vi "ADC_and_DAC.vi"(1 "ADS Mode In":i32=1 min=1 max=6 step=1, 2 "Board address":i32=4660 format="%x") -> (0 "ADS Mode Out":i32)   [LabVIEW 2011]
doc: "This VI is a pop-up window that allows full access to the MUX, DAC, and A/D converter. This should be included with all USB-DAQ applications as a debug tool. You can also look through the software as an example of how to configure the MUX, DAC, and A/D converter."
panel:
  out "ADC 2":string
  out "ADC 1":string
  in  "User Ref Voltage":dbl
  in  "Connect I Loop Readback":bool
  in  "ADS2- MUX":enum32{"Open", "Dac C", "GND"}(radio)
  in  "ADS2+ MUX":enum32{"Open", "Dac D", "GND"}(radio)
  in  "ADS1- MUX":enum32{"Open", "Dac A", "GND"}(radio)
  in  "ADS1+ MUX":enum32{"Open", "Dac B", "GND"}(radio)
  in  "ReadADC_2":bool
  in  "ReadADC_1":bool
  in  "Write_DAC_D":bool
  in  "Write_DAC_C":bool
  in  "Write_DAC_B":bool
  in  "Write_DAC_A":bool
  in  "DAC_D":dbl=0.017 min=0.017 max=5.0
  in  "DAC_C":dbl=0.017 min=0.017 max=5.0
  in  "DAC_B":dbl=0.017 min=0.017 max=5.0
  in  "DAC_A":dbl=0.017 min=0.017 max=5.0
  in  "ADC Config":T1(radio)
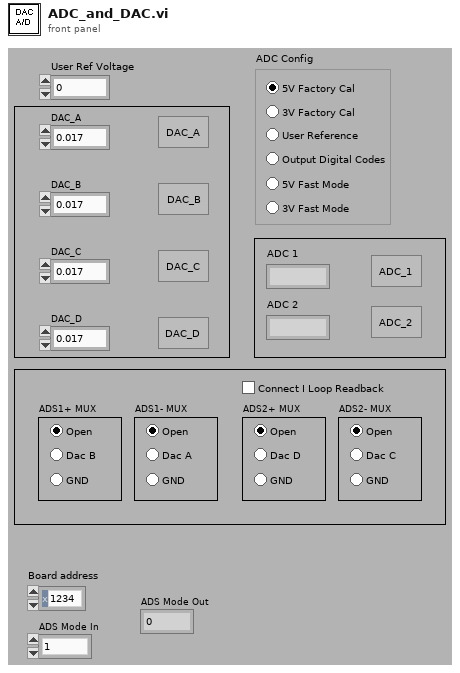
[diagram p1: front panel]
types:
  T1 = enum32{"5V Factory Cal", "3V Factory Cal", "User Reference", "Output Digital Codes", "5V Fast Mode", "3V Fast Mode"}
  T2 = enum32{"Invalid", "Standard", "Closed", "Hidden", "Minimized", "Maximized"}
  T3 = enum16{"Always On", "Always Off", "Off While Running"}
  T4 = enum32{"invalid app kind", "Development System", "Run Time System", "Student Edition", "Embedded LabVIEW", "Evaluation", "Custom"}
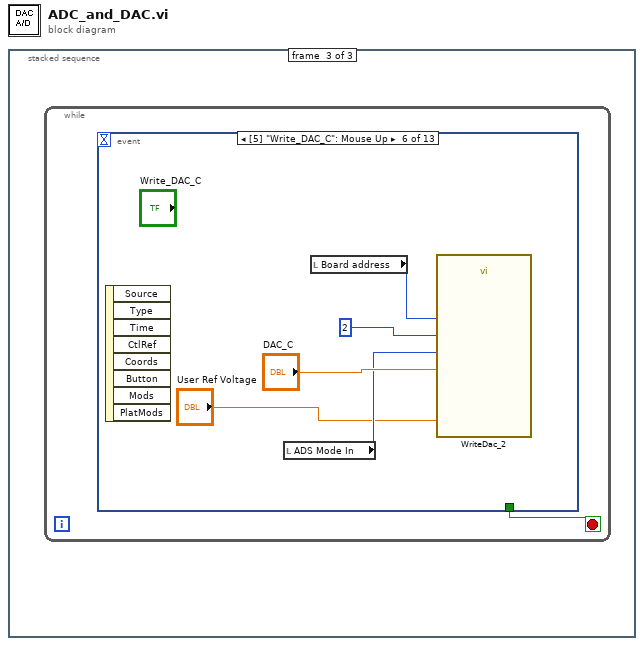
[diagram p0: block diagram]
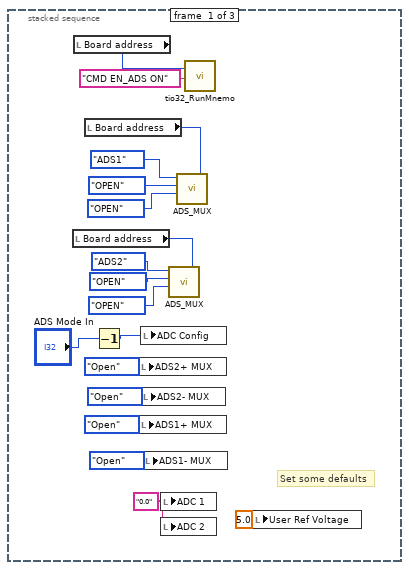
[diagram p2: hidden frame]
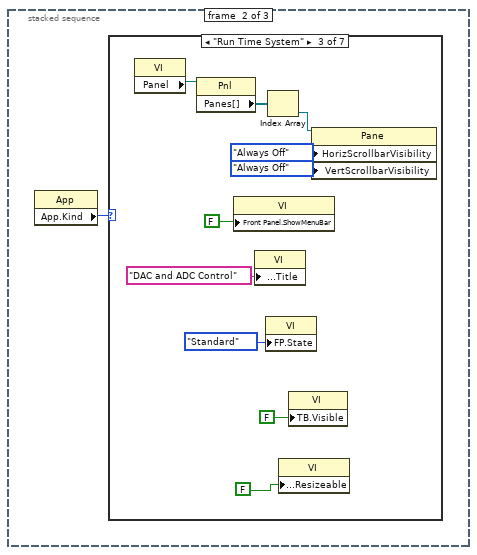
[diagram p3: hidden frame]
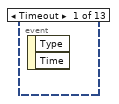
[diagram p10: hidden frame]
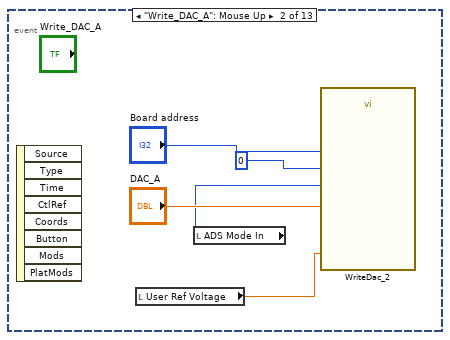
[diagram p11: hidden frame]
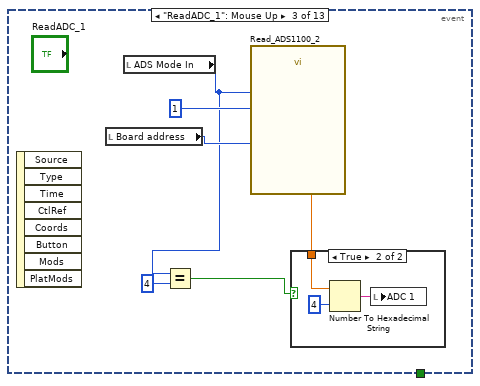
[diagram p12: hidden frame]
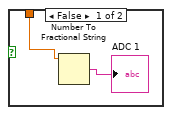
[diagram p13: hidden frame]
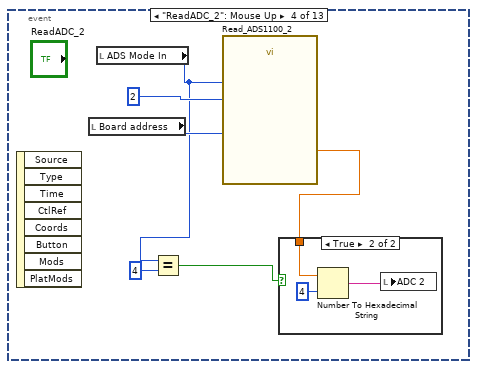
[diagram p14: hidden frame]
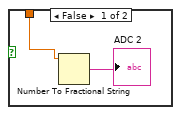
[diagram p15: hidden frame]
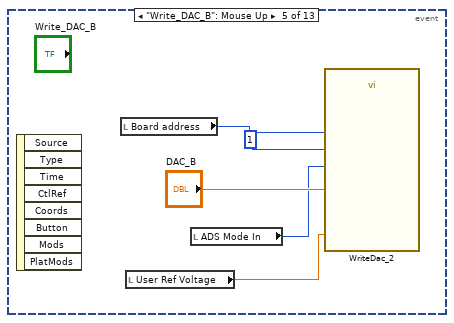
[diagram p16: hidden frame]
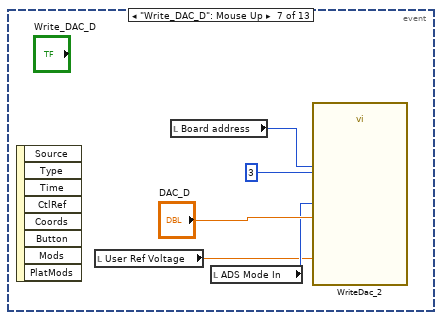
[diagram p17: hidden frame]
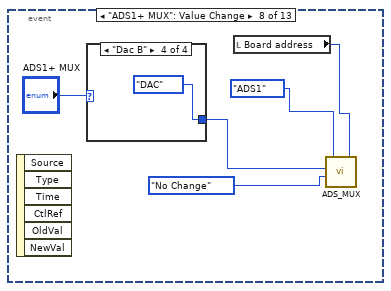
[diagram p18: hidden frame]
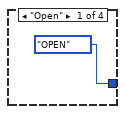
[diagram p19: hidden frame]
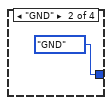
[diagram p20: hidden frame]
diagram:
  n1 = stacked-sequence {
    frame #0 {
      w2 = "0.0" ("ADC 1")
      # "Set some defaults"
      n2 = local read "Board address"() -> (w8:i32)
      n3 = local read "Board address"() -> (w18:i32)
      n4 = local read "Board address"() -> (w9:i32)
      n5 = Decrement(x="ADS Mode In") -> (x-1=w3:i32)
      n6 = local write "ADS2+ MUX"(enum32{"Open", "Dac D", "GND"}."Open" ("ADS2+ MUX")) -> ()
      n7 = local write "ADS1+ MUX"(enum32{"Open", "Dac B", "GND"}."Open" ("ADS1+ MUX")) -> ()
      n8 = local write "ADC Config"(w3) -> ()
      n9 = local write "ADS2- MUX"(enum32{"Open", "Dac C", "GND"}."Open" ("ADS2- MUX")) -> ()
      n10 = local write "ADS1- MUX"(enum32{"Open", "Dac A", "GND"}."Open" ("ADS1- MUX")) -> ()
      n11 = local write "ADC 1"(w2) -> ()
      n12 = local write "ADC 2"(w2) -> ()
      n13 = call "ADS_MUX.vi"("Board address"=w8, "In Neg"=enum16{"OPEN", "GND", "DAC", "No Change"}."OPEN", "In Pos"=enum16{"OPEN", "GND", "DAC", "No Change"}."OPEN", "Mux Num"=enum16{"ADS1", "ADS2"}."ADS2") -> ()  [unwired: 1 in, 1 out]
      n14 = call "ADS_MUX.vi"("Board address"=w9, "In Neg"=enum16{"OPEN", "GND", "DAC", "No Change"}."OPEN", "In Pos"=enum16{"OPEN", "GND", "DAC", "No Change"}."OPEN", "Mux Num"=enum16{"ADS1", "ADS2"}."ADS1") -> ()  [unwired: 1 in, 1 out]
      n15 = call "tio32_RunMnemo.vi"("Device address"=w18, "command string"="CMD EN_ADS ON") -> ()  [unwired: 7 in, 11 out]
      n16 = local write "User Ref Voltage"(5.0 ("User Ref Voltage")) -> ()
    }
    frame #1 {
      n17 = property class="App"() -> ("App.Kind"=w19:T4)  [unwired: 2 in, 2 out]
      n18 = case shown="\"Run Time System\"" w19 {
        frame "invalid app kind", Default {
        }
        frame "Development System" {
        }
        frame "Run Time System" {
          n19 = property class="VI"() -> ("Panel"=w29:refnum<vi>)  [unwired: 2 in, 2 out]
          n20 = property class="Pnl"(reference=w29) -> ("Panes[]"=w28:refnum<vi>[])  [unwired: 1 in, 2 out]
          n21 = property class="VI"("Front Panel.ShowMenuBar"=FALSE ("Front Panel Window:Show Menu Bar")) -> ()  [unwired: 2 in, 2 out]
          n22 = property class="VI"("Front Panel.Title"="DAC and ADC Control" ("Front Panel Window:Title")) -> ()  [unwired: 2 in, 2 out]
          n23 = property class="VI"("FP.State"=T2."Standard" ("Front Panel Window:State")) -> ()  [unwired: 2 in, 2 out]
          n24 = Index Array(array=w28) -> (element=w27:refnum<vi>)  [unwired: 1 in]
          n25 = property class="VI"("Front Panel.Resizeable"=FALSE ("Front Panel Window:Resizeable")) -> ()  [unwired: 2 in, 2 out]
          n26 = property class="VI"("TB.Visible"=FALSE ("Front Panel Window:Resizeable")) -> ()  [unwired: 2 in, 2 out]
          n27 = property class="Pane"(reference=w27, "HorizScrollbarVisibility"=T3."Always Off" ("Horizontal Scrollbar Visibility"), "VertScrollbarVisibility"=T3."Always Off" ("Vertical Scrollbar Visibility")) -> ()  [unwired: 1 in, 2 out]
        }
        frame "Student Edition" {
        }
        frame "Embedded LabVIEW" {
        }
        frame "Evaluation" {
        }
        frame "Custom" {
        }
      }
    }
    frame #2 {
      n28 = while {
        stop <- w30 stop-if-true
        n29 = event shown="[5] \"Write_DAC_C\": Mouse Up" {
          selector: _ -> [_ _ _ _ _ _ _ _ _ _ _ _ _]
          dyn-events: _ -> [_ _ _ _ _ _ _ _ _ _ _ _ _]
          timeout: _ -> [_ _ _ _ _ _ _ _ _ _ _ _ _]
          tunnel: [_ _ _ _ _ _ _ _ _ _ _ _ w116] -> w30
          event Timeout {
            n30 = event-data() -> ()  [unwired: 1 in, 2 out]
          }
          event "Write_DAC_A": Mouse Up {
            n31 = event-data() -> ()  [unwired: 1 in, 8 out]
            n32 = local read "User Ref Voltage"() -> (w31:dbl)
            n33 = local read "ADS Mode In"() -> (w32:i32)
            n34 = call "WriteDac_2.vi"("ref"=w31, "value"="DAC_A", "mode"=w32, "DAC number"=0, "Board address"="Board address") -> ()  [unwired: 4 in, 1 out]
          }
          event "ReadADC_1": Mouse Up {
            n35 = event-data() -> ()  [unwired: 1 in, 8 out]
            n36 = local read "Board address"() -> (w41:i32)
            n37 = local read "ADS Mode In"() -> (w38:i32)
            n38 = Equal?(x=w38, y=4) -> (x = y?=w36:bool)
            n39 = call "Read_ADS1100_2.vi"("USB DAQ Address"=w41, "ADS Mode"=w38, "ADS number"=1 ("mode")) -> ("ADC"=w39:dbl)  [unwired: 1 in, 1 out]
            n40 = case shown="True" w36 {
              tunnel: w39 -> [w43 w46]
              frame False {
                n41 = Number To Fractional String(number=w43) -> (F-format string=→"ADC 1":string)  [unwired: 3 in]
              }
              frame True {
                n42 = Number To Hexadecimal String(1:i16 4 ("width (-)"), 2:w46) -> (0:w45:string)
                n43 = local write "ADC 1"(w45) -> ()
              }
            }
          }
          event "ReadADC_2": Mouse Up {
            n44 = event-data() -> ()  [unwired: 1 in, 8 out]
            n45 = local read "Board address"() -> (w51:i32)
            n46 = local read "ADS Mode In"() -> (w47:i32)
            n47 = Equal?(x=w47, y=4) -> (x = y?=w49:bool)
            n48 = call "Read_ADS1100_2.vi"("USB DAQ Address"=w51, "ADS Mode"=w47, "ADS number"=2) -> ("ADC"=w48:dbl)  [unwired: 1 in, 1 out]
            n49 = case shown="True" w49 {
              tunnel: w48 -> [w54 w57]
              frame False {
                n50 = Number To Fractional String(number=w54) -> (F-format string=→"ADC 2":string)  [unwired: 3 in]
              }
              frame True {
                n51 = Number To Hexadecimal String(1:i16 4 ("width (-)"), 2:w57) -> (0:w55:string)
                n52 = local write "ADC 2"(w55) -> ()
              }
            }
          }
          event "Write_DAC_B": Mouse Up {
            n53 = event-data() -> ()  [unwired: 1 in, 8 out]
            n54 = local read "Board address"() -> (w62:i32)
            n55 = local read "User Ref Voltage"() -> (w58:dbl)
            n56 = local read "ADS Mode In"() -> (w59:i32)
            n57 = call "WriteDac_2.vi"("ref"=w58, "value"="DAC_B", "mode"=w59, "DAC number"=1, "Board address"=w62) -> ()  [unwired: 4 in, 1 out]
          }
          event "Write_DAC_C": Mouse Up {
            n58 = event-data() -> ()  [unwired: 1 in, 8 out]
            n59 = local read "ADS Mode In"() -> (w64:i32)
            n60 = local read "Board address"() -> (w67:i32)
            n61 = call "WriteDac_2.vi"("ref"="User Ref Voltage", "value"="DAC_C", "mode"=w64, "DAC number"=2, "Board address"=w67) -> ()  [unwired: 4 in, 1 out]
          }
          event "Write_DAC_D": Mouse Up {
            n62 = event-data() -> ()  [unwired: 1 in, 8 out]
            n63 = local read "User Ref Voltage"() -> (w68:dbl)
            n64 = local read "Board address"() -> (w70:i32)
            n65 = local read "ADS Mode In"() -> (w69:i32)
            n66 = call "WriteDac_2.vi"("ref"=w68, "value"="DAC_D", "mode"=w69, "DAC number"=3, "Board address"=w70) -> ()  [unwired: 4 in, 1 out]
          }
          event "ADS1+ MUX": Value Change {
            n67 = event-data() -> ()  [unwired: 1 in, 6 out]
            n68 = case shown="\"Dac B\"" "ADS1+ MUX" {
              tunnel: [enum16{"OPEN", "GND", "DAC", "No Change"}."OPEN" ("In Pos") enum16{"OPEN", "GND", "DAC", "No Change"}."GND" ("In Pos") enum16{"OPEN", "GND", "DAC", "No Change"}."No Change" ("In Pos") enum16{"OPEN", "GND", "DAC", "No Change"}."DAC" ("In Pos")] -> w74
              frame "Open" {
              }
              frame "GND" {
              }
              frame Default {
              }
              frame "Dac B" {
              }
            }
            n69 = local read "Board address"() -> (w76:i32)
            n70 = call "ADS_MUX.vi"("Board address"=w76, "In Neg"=enum16{"OPEN", "GND", "DAC", "No Change"}."No Change", "In Pos"=w74, "Mux Num"=enum16{"ADS1", "ADS2"}."ADS1" ("Mux")) -> ()  [unwired: 1 in, 1 out]
          }
          event "ADS1- MUX": Value Change {
            n71 = event-data() -> ()  [unwired: 1 in, 6 out]
            n72 = case shown="\"GND\"" "ADS1- MUX" {
              tunnel: [enum16{"OPEN", "GND", "DAC", "No Change"}."OPEN" ("In Neg") enum16{"OPEN", "GND", "DAC", "No Change"}."DAC" ("In Neg") enum16{"OPEN", "GND", "DAC", "No Change"}."GND" ("In Neg") enum16{"OPEN", "GND", "DAC", "No Change"}."No Change" ("In Neg")] -> w82
              frame "Open" {
              }
              frame "Dac A" {
              }
              frame "GND" {
              }
              frame Default {
              }
            }
            n73 = local read "Board address"() -> (w86:i32)
            n74 = call "ADS_MUX.vi"("Board address"=w86, "In Neg"=w82, "In Pos"=enum16{"OPEN", "GND", "DAC", "No Change"}."No Change", "Mux Num"=enum16{"ADS1", "ADS2"}."ADS1" ("Mux")) -> ()  [unwired: 1 in, 1 out]
          }
          event "ADS2+ MUX": Value Change {
            n75 = event-data() -> ()  [unwired: 1 in, 6 out]
            n76 = case shown="Default" "ADS2+ MUX" {
              tunnel: [enum16{"OPEN", "GND", "DAC", "No Change"}."OPEN" ("In Pos") enum16{"OPEN", "GND", "DAC", "No Change"}."DAC" ("In Pos") enum16{"OPEN", "GND", "DAC", "No Change"}."GND" ("In Pos") enum16{"OPEN", "GND", "DAC", "No Change"}."No Change" ("In Pos")] -> w92
              frame "Open" {
              }
              frame "Dac D" {
              }
              frame "GND" {
              }
              frame Default {
              }
            }
            n77 = local read "Board address"() -> (w94:i32)
            n78 = call "ADS_MUX.vi"("Board address"=w94, "In Neg"=enum16{"OPEN", "GND", "DAC", "No Change"}."No Change", "In Pos"=w92, "Mux Num"=enum16{"ADS1", "ADS2"}."ADS2") -> ()  [unwired: 1 in, 1 out]
          }
          event "ADS2- MUX": Value Change {
            n79 = event-data() -> ()  [unwired: 1 in, 6 out]
            n80 = case shown="\"Dac C\"" "ADS2- MUX" {
              tunnel: [enum16{"OPEN", "GND", "DAC", "No Change"}."OPEN" ("In Neg") enum16{"OPEN", "GND", "DAC", "No Change"}."GND" ("In Neg") enum16{"OPEN", "GND", "DAC", "No Change"}."DAC" ("In Neg") enum16{"OPEN", "GND", "DAC", "No Change"}."No Change" ("In Neg")] -> w102
              frame "Open" {
              }
              frame "GND" {
              }
              frame "Dac C" {
              }
              frame Default {
              }
            }
            n81 = local read "Board address"() -> (w103:i32)
            n82 = call "ADS_MUX.vi"("Board address"=w103, "In Neg"=w102, "In Pos"=enum16{"OPEN", "GND", "DAC", "No Change"}."No Change", "Mux Num"=enum16{"ADS1", "ADS2"}."ADS2") -> ()  [unwired: 1 in, 1 out]
          }
          event "ADC Config": Value Change {
            n83 = event-data() -> ()  [unwired: 1 in, 6 out]
            n84 = case shown="\"Output Digital Codes\"" "ADC Config" {
              frame "5V Factory Cal", Default {
                n85 = local write "ADS Mode In"(1 ("ADS Mode In")) -> ()
              }
              frame "3V Factory Cal" {
                n86 = local write "ADS Mode In"(2 ("ADS Mode In")) -> ()
              }
              frame "User Reference" {
                n87 = local write "ADS Mode In"(3 ("ADS Mode In")) -> ()
              }
              frame "Output Digital Codes" {
                n88 = local write "ADS Mode In"(4 ("ADS Mode In")) -> ()
              }
              frame "5V Fast Mode" {
                n89 = local write "ADS Mode In"(5 ("ADS Mode In")) -> ()
              }
              frame "3V Fast Mode" {
                n90 = local write "ADS Mode In"(6 ("ADS Mode In")) -> ()
              }
            }
          }
          event Panel Close {
            n91 = event-data() -> ()  [unwired: 1 in, 4 out]
            n92 = flat-sequence {
              tunnel: [TRUE] -> w116
              frame #0 {
                n93 = local read "ADS Mode In"() -> (→"ADS Mode Out":i32)
              }
              frame #1 {
              }
            }
          }
        }
      }
    }
  }
